vi "sub_cumsum.vi"(11 "in mat":T1) -> (3 "cumsum":dbl[](array[numeric]))   [LabVIEW 2019]
uses:
  <vilib>/Analysis/Matrix/Datatypes/RealMatrix.ctl
  <vilib>/Analysis/Matrix/NI_Matrix.lvlib
panel:
  out "subarray":dbl[](array[numeric])
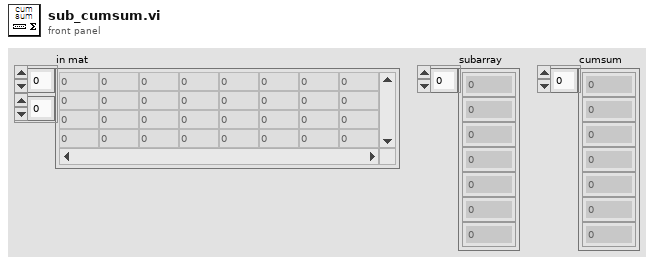
[diagram p1: front panel]
types:
  T1 = typedef "NI_Matrix.lvlib/RealMatrix.ctl" = dbl[][]
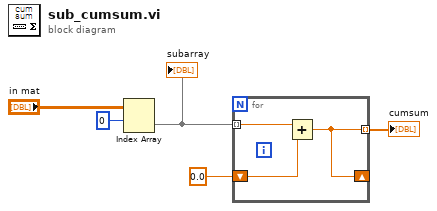
[diagram p0: block diagram]
diagram:
  n1 = Index Array(array="in mat", index (row)=0) -> (element=w1:dbl[])  [unwired: 1 in]
  "subarray" <- w1
  n2 = for {
    shift-right: [w7] -> _
    shift-left: 0.0 -> [w8]
    tunnel: [w7] -> w3 mode=indexing
    tunnel: w1 -> [w6] mode=indexing
    n3 = Add(x=w6, y=w8) -> (x+y=w7:dbl)
  }
  "cumsum" <- w3
